vi "SubVI_ScaleNativeTester.vi"(10 "forward input":dbl(slide) scale=-1.0..1.0, 11 "left input":dbl(slide) scale=1.0..-1.0) -> (2 "Right Predicted":dbl(slide) scale=-18000.0..18000.0, 3 "Left Predicted":dbl(slide) scale=-18000.0..18000.0)   [LabVIEW 2017]
panel:
  in  "Scale Turn":dbl=36000.0 format="%#_13g"
  in  "Scale Drive":dbl=18000.0 format="%#_13g"
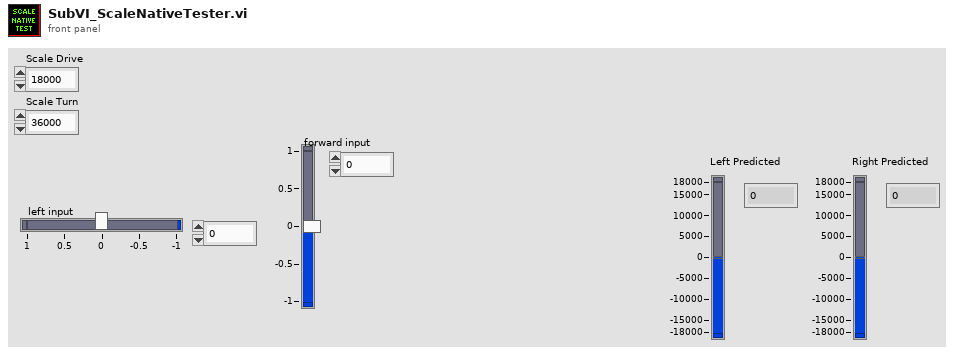
[diagram p1: front panel]
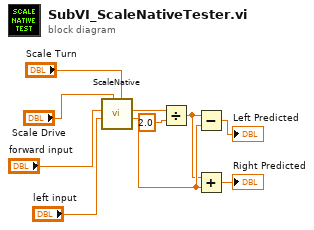
[diagram p0: block diagram]
diagram:
  n1 = call "ScaleNative.vi"("Scale Turn"="Scale Turn", "Scale Drive"="Scale Drive", "Left"="left input", "Forward"="forward input") -> ("CounterClock Scaled"=w4:dbl, "Forward Scaled"=w3:dbl)  [unwired: 6 in]
  n2 = Divide(x=w3, y=2.0) -> (x/y=w1:dbl)
  n3 = Subtract(x=w1, y=w4) -> (x-y=→"Left Predicted":dbl)
  n4 = Add(x=w1, y=w4) -> (x+y=→"Right Predicted":dbl)
